vi "Main.vi"() -> ()   [LabVIEW 2018]
doc: "The myRIO Project template acquires acceleration data from the onboard accelerometer and displays the changes of acceleration values in a waveform chart."
uses:
  <vilib>/Platform/TimedLoop/XDataNode/timing_clust.ctl
  <vilib>/Platform/TimedLoop/XDataNode/nitl_modes.ctl
  <vilib>/Platform/TimedLoop/XDataNode/wakeup.ctl
  <vilib>/myRIO/Instrument Drivers/Onboard IO/DIO/typedefs/DIO Reference.ctl
  <vilib>/myRIO/Common/Instrument Driver Framework/Utilities/typedefs/myRIO Generic Hardware Reference.ctl
  <vilib>/myRIO/Common/Instrument Driver Framework/Utilities/typedefs/Hardware Version Enum.ctl
  <vilib>/myRIO/Common/Instrument Driver Framework/Utilities/typedefs/myRIO v1.0 Reference.ctl
  <vilib>/myRIO/Common/Instrument Driver Framework/Utilities/typedefs/Generic FPGA Reference.ctl
  <vilib>/myRIO/Common/Instrument Driver Framework/myRIO v1.0/DIO/typedefs/DIO Channels List.ctl
  <vilib>/myRIO/Common/Instrument Driver Framework/myRIO v1.0/DIO/typedefs/DIO Channels Enum.ctl
  <vilib>/userdefined/High Color/nirio_resource_hc.ctl
  <vilib>/myRIO/Instrument Drivers/Onboard IO/AI/typedefs/AI Reference.ctl
  <vilib>/myRIO/Common/Instrument Driver Framework/myRIO v1.0/AI/typedefs/AI Channels List.ctl
  <vilib>/myRIO/Common/Instrument Driver Framework/myRIO v1.0/AI/typedefs/AI Channels Enum.ctl
  <vilib>/myRIO/Common/Instrument Driver Framework/Utilities/typedefs/Analog Scaling Constants List.ctl
  <vilib>/myRIO/Common/Instrument Driver Framework/Utilities/typedefs/Analog Scaling Constants.ctl
  <vilib>/myRIO/Instrument Drivers/Onboard IO/AO/typedefs/AO Reference.ctl
  <vilib>/myRIO/Common/Instrument Driver Framework/myRIO v1.0/AO/typedefs/AO Channels List.ctl
  <vilib>/myRIO/Common/Instrument Driver Framework/myRIO v1.0/AO/typedefs/AO Channels Enum.ctl
  <vilib>/myRIO/Common/Instrument Driver Framework/Utilities/vis/Is FPGA Ref Available.vi
  <vilib>/myRIO/Common/Instrument Driver Framework/myRIO v1.0/DIO/vis/myRIO v1.1 Open DIO.vi
  <vilib>/myRIO/Instrument Drivers/Onboard IO/DIO/vis/Read.vi
  <vilib>/myRIO/Instrument Drivers/Onboard IO/DIO/vis/Write.vi
  <vilib>/myRIO/Common/Instrument Driver Framework/myRIO v1.0/AI/vis/myRIO v1.1 Open AI.vi
  <vilib>/myRIO/Instrument Drivers/Onboard IO/AI/vis/Read.vi
  <vilib>/myRIO/Common/Instrument Driver Framework/myRIO v1.0/AO/vis/myRIO v1.1 Open AO.vi
  <vilib>/myRIO/Instrument Drivers/Onboard IO/AO/vis/Write.vi
  <vilib>/myRIO/Common/Instrument Driver Framework/Utilities/vis/Validate Channels.vi
  <vilib>/myRIO/Common/Instrument Driver Framework/myRIO v1.0/DIO/vis/myRIO v1.0 Reserve DIO.vi
  <vilib>/myRIO/Common/Instrument Driver Framework/myRIO v1.0/AI/vis/myRIO v1.0 Reserve AI.vi
  <vilib>/myRIO/Common/Instrument Driver Framework/myRIO v1.0/AO/vis/myRIO v1.0 Reserve AO.vi
  <vilib>/myRIO/Common/Instrument Driver Framework/myRIO v1.0/Resource Manager/vis/myRIO v1.0 Reserve Channel List.vi
  <vilib>/myRIO/Common/Instrument Driver Framework/myRIO v1.0/DIO/vis/myRIO v1.0 Build MUX Configuration DIO.vi
  <vilib>/myRIO/Common/Instrument Driver Framework/myRIO v1.0/AI/vis/myRIO v1.0 Build MUX Configuration AI.vi
  <vilib>/myRIO/Common/Instrument Driver Framework/myRIO v1.0/AO/vis/myRIO v1.0 Build MUX Configuration AO.vi
  <vilib>/myRIO/Common/Instrument Driver Framework/myRIO v1.0/Resource Manager/vis/myRIO v1.0 Reserve Channel.vi
  <vilib>/myRIO/Common/Instrument Driver Framework/myRIO v1.0/Resource Manager/vis/myRIO v1.0 Unreserve Channel.vi
  <vilib>/myRIO/Common/Instrument Driver Framework/myRIO v1.0/Resource Manager/vis/myRIO v1.0 Create Configuration List.vi
  <vilib>/myRIO/Common/Instrument Driver Framework/myRIO v1.0/Resource Manager/vis/myRIO v1.0 Build Mutex Name.vi
  <vilib>/Utility/VariantDataType/GetNumericInfo.vi
  <vilib>/Utility/error.llb/Error Cluster From Error Code.vi
  <vilib>/myRIO/Common/Instrument Driver Framework/myRIO v1.0/myRIO v1.1 Open.vi
  <vilib>/myRIO/Common/Instrument Driver Framework/Utilities/vis/IO Manager.vi
  <vilib>/myRIO/Common/Instrument Driver Framework/Utilities/vis/Configuration Manager.vi
  <vilib>/myRIO/Common/Instrument Driver Framework/myRIO v1.0/Resource Manager/vis/myRIO v1.0 Configure IO.vi
  <vilib>/myRIO/Common/Instrument Driver Framework/myRIO v1.0/myRIO v1.0 Close.vi
  <vilib>/myRIO/Common/Instrument Driver Framework/myRIO v1.0/DIO/vis/myRIO v1.0 Write DIO.vi
  <vilib>/myRIO/Common/Instrument Driver Framework/myRIO v1.0/AI/vis/myRIO v1.0 Get Scaling Constants AI.vi
  <vilib>/myRIO/Common/Instrument Driver Framework/myRIO v1.0/AI/vis/myRIO v1.0 Read AI.vi
  <vilib>/functionblocks/Bistables/SR Bistable/SR Bistable.vi
  <vilib>/myRIO/Common/Instrument Driver Framework/myRIO v1.0/AO/vis/myRIO v1.0 Get Scaling Constants AO.vi
  <vilib>/myRIO/Common/Instrument Driver Framework/myRIO v1.0/AO/vis/myRIO v1.0 Write AO.vi
  <vilib>/functionblocks/Counter/Pulse Timer/Pulse Timer.vi
  <vilib>/myRIO/Common/Instrument Driver Framework/myRIO v1.0/DIO/vis/myRIO v1.0 Read DIO.vi
  <vilib>/myRIO/Express VI/Onboard IO/DO/DO Express VI.xnode
  <vilib>/myRIO/Instrument Drivers/Onboard IO/DIO/vis/myRIO DIO Open.xnode
  <vilib>/Platform/TimedLoop/XDataNode/XDataNode.xnode
  <vilib>/myRIO/Express VI/Onboard IO/AI/AI Express VI.xnode
  <vilib>/myRIO/Instrument Drivers/Onboard IO/AI/vis/myRIO AI Open.xnode
  <vilib>/functionblocks/FB Core/FB Core.xnode
  <vilib>/myRIO/Express VI/Onboard Devices/LED/LED Express VI.xnode
  <vilib>/myRIO/Express VI/Onboard IO/AO/AO Express VI.xnode
  <vilib>/myRIO/Instrument Drivers/Onboard IO/AO/vis/myRIO AO Open.xnode
  <vilib>/myRIO/Express VI/Onboard IO/DI/DI Express VI.xnode
  <vilib>/myRIO/Express VI/Onboard Devices/Button/Button Express VI.xnode
  <vilib>/myRIO/Instrument Drivers/Onboard IO/DIO/DIO.lvlib
  <vilib>/myRIO/Instrument Drivers/Onboard IO/AI/AI.lvlib
  <vilib>/myRIO/Instrument Drivers/Onboard IO/AO/AO.lvlib
  <vilib>/functionblocks/NI_FunctionBlock Libraries.lvlib
  <vilib>/Platform/TimedLoop/XDataNode/XDNodeRunTimeDep.lvlib
panel:
  out "Pump out":bool
  out "RTD Status LED":bool
  out "RFE Indicator":bool
  out "AIR + Boolean":bool
  out "AIR +(A9)":dbl
  out "RTD Button":bool
  out "RTD Brake":bool
  out "EN Indicator":bool
  out "RTD Buzzer":bool
  in  "Buzzer test":bool
  in  "RTD Brake Test":bool
  in  "RFE  Test":bool
  in  "EN Test":bool
  out "APPS1 (V) Input (B/AI0 (Pin 3))":dbl
  out "APPS2 Scaled Up (V)":dbl
  out "APPS1 Scaled Up (V)":dbl
  out "APPS2 (V) Input (B/AI1 (Pin 5))":dbl
  out "APPS fault":bool
  out "APPS2 %":dbl
  out "APPS1 %":dbl
  out "APPS Output (V)":dbl
  out "APPS output %":dbl
  out "Accelaration":dbl(knob) scale=0.0..100.0
  out "APPS1":dbl(knob) scale=0.0..100.0
  out "APPS2":dbl(knob) scale=0.0..100.0
  out "APPS pedal travel %":dbl
  out "RTD Brake 2":bool
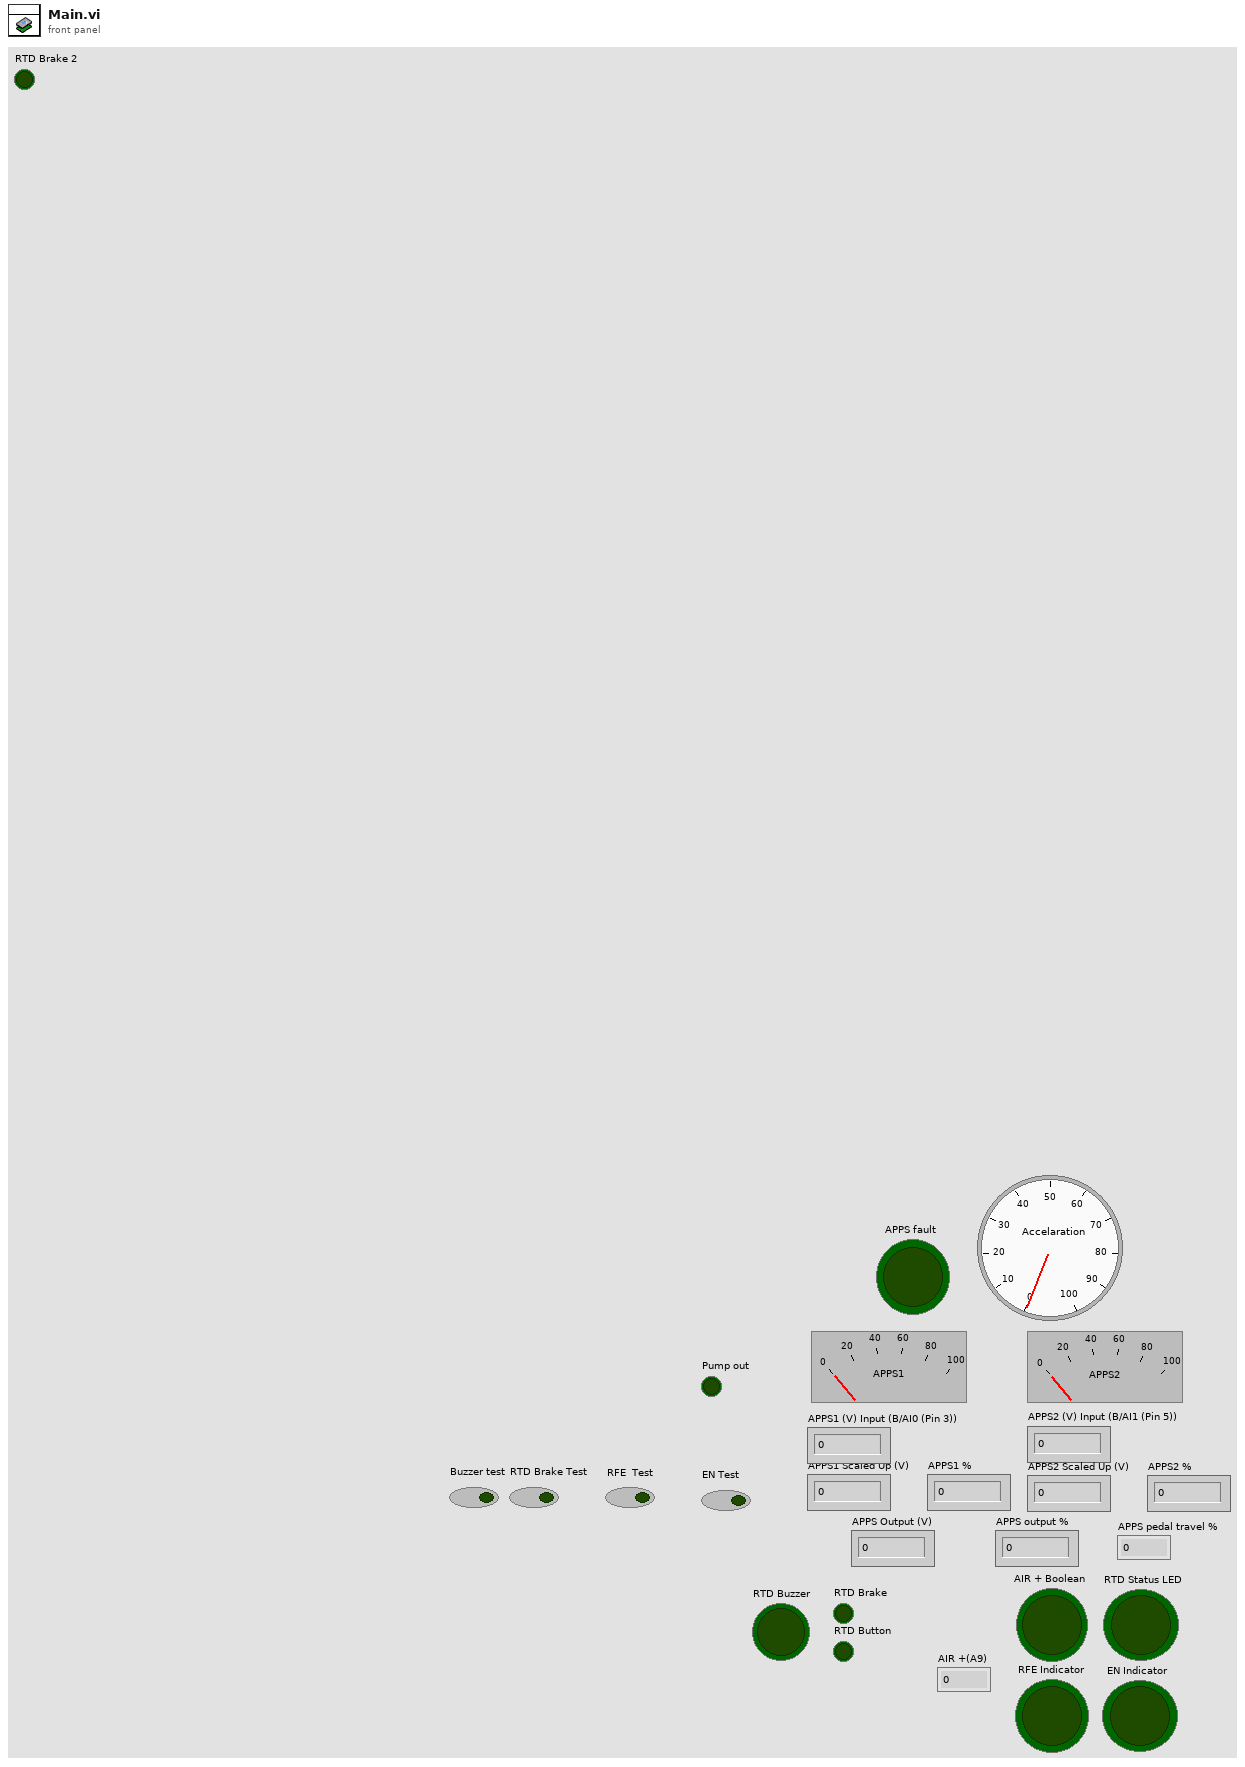
[diagram p1: front panel]
types:
  T1 = typedef "XDNodeRunTimeDep.lvlib/timing_clust.ctl" = cluster{"Expected End [f-1]":u64, "Actual End [f-1]":u64, "Finished Late? [f-1]":bool, "Expected End [i-1]":u64, "Actual End [i-1]":u64, "Finished Late? [i-1]":bool, "Expected Start [i]":u64, "Actual Start [i]":u64, "Expected Start [f]":u64, "Actual Start [f]":u64, "Source Name":string, "Structure Name":string, "Period":i64, "Deadline":i64, "Offset":i64, "Start":i64, "Priority":i32, "Timeout":i32, "Mode":T2, "Wakeup Reason":T3, "Error":errorcluster, "Source Type":string, "Secondary Source Type":string, "Global End Time":u64, "Global Start Time":u64, "Frame Duration":u64, "Iteration Duration":u64, "Assigned CPU":i32, "I/O Scan Engine Mode":u32}
  T2 = typedef "XDNodeRunTimeDep.lvlib/nitl_modes.ctl" = enum32{"No Change", "Process missed periods, maintain original phase", "Discard missed periods, maintain original phase", "Process missed periods, ignore original phase", "Discard missed periods, ignore original phase"}
  T3 = typedef "XDNodeRunTimeDep.lvlib/wakeup.ctl" = enum32{"Normal", "Aborted", "Asynchronous wakeup", "Timing source error", "Timed loop error", "Timeout"}
  T4 = typedef "DIO.lvlib/DIO Reference.ctl" = cluster{"myRIO Reference":T5, "DIO Channels List":T9}
  T5 = typedef "myRIO Generic Hardware Reference.ctl" = cluster{"myRIO Model":T6, "myRIO Hardware Reference":T7}
  T6 = typedef "Hardware Version Enum.ctl" = enum16{"Unknown", "myRIO-1900", "myRIO-1950", "roboRIO", "NI ELVIS RIO CM", "ELVIS III"}
  T7 = typedef "myRIO v1.0 Reference.ctl" = cluster{"Generic FPGA Reference":T8, "Allow multiple opens":bool}
  T8 = typedef "Generic FPGA Reference.ctl" = refnum<k20>
  T9 = typedef "DIO Channels List.ctl" = T10[]
  T10 = typedef "DIO Channels Enum.ctl" = enum16{"Not Connected", "C/DIO0", "C/DIO1", "C/DIO2", "C/DIO3", "C/DIO4", "C/DIO5", "C/DIO6", "C/DIO7", "A/DIO0", "A/DIO1", "A/DIO2", "A/DIO3", "A/DIO4", "A/DIO5", "A/DIO6", "A/DIO7", "A/DIO8", "A/DIO9", "A/DIO10", "A/DIO11", "A/DIO12", "A/DIO13", "A/DIO14", "A/DIO15", "A/DIO16", "A/DIO17", "A/DIO18", "A/DIO19", "B/DIO0", "B/DIO1", "B/DIO2", "B/DIO3", "B/DIO4", "B/DIO5", "B/DIO6", "B/DIO7", "B/DIO8", "B/DIO9", "B/DIO10", "B/DIO11", "B/DIO12", "B/DIO13", "B/DIO14", "B/DIO15", "B/DIO16", "B/DIO17", "B/DIO18", "B/DIO19", "LED0", "LED1", "LED2", "LED3", "Button0", "DIO/DIO0", "DIO/DIO1", "DIO/DIO2", "DIO/DIO3", "DIO/DIO4", "DIO/DIO5", "DIO/DIO6", "DIO/DIO7", "DIO/DIO8", "DIO/DIO9", "SPI/CS0", "SPI/CS1", "SPI/CS2", "SPI/CS3", "LED RADIO (Green)", "LED RADIO (Red)", "LED COMM (Green)", "LED COMM (Red)", "LED MODE (Green)", "LED MODE (Red)"}
  T11 = typedef "nirio_resource_hc.ctl" = tag
  T12 = typedef "AO.lvlib/AO Reference.ctl" = cluster{"myRIO Reference":T5, "AO Channel List":T13, "AO Scaling Constant List":T15}
  T13 = typedef "AO Channels List.ctl" = T14[]
  T14 = typedef "AO Channels Enum.ctl" = enum16{"Not Connected", "AudioOut/Left", "AudioOut/Right", "C/AO0", "C/AO1", "A/AO0", "A/AO1", "B/AO0", "B/AO1"}
  T15 = typedef "Analog Scaling Constants List.ctl" = T16[]
  T16 = typedef "Analog Scaling Constants.ctl" = cluster{"LSB Weight (Volts)":dbl, "Offset (Volts)":dbl, "Signed?":bool}
  T17 = typedef "AI.lvlib/AI Reference.ctl" = cluster{"myRIO Reference":T5, "AI Channels List":T18, "AI Scaling Constants List":T15}
  T18 = typedef "AI Channels List.ctl" = T19[]
  T19 = typedef "AI Channels Enum.ctl" = enum16{"Not Connected", "AudioIn/Left", "AudioIn/Right", "C/AI0", "C/AI1", "A/AI0", "A/AI1", "A/AI2", "A/AI3", "A/AI4", "A/AI5", "A/AI6", "A/AI7", "B/AI0", "B/AI1", "B/AI2", "B/AI3", "B/AI4", "B/AI5", "B/AI6", "B/AI7", "AI/AI0", "AI/AI1", "AI/AI2", "AI/AI3", "A/AI0 (DIFF)", "A/AI1 (DIFF)", "A/AI2 (DIFF)", "A/AI3 (DIFF)", "B/AI0 (DIFF)", "B/AI1 (DIFF)", "B/AI2 (DIFF)", "B/AI3 (DIFF)"}
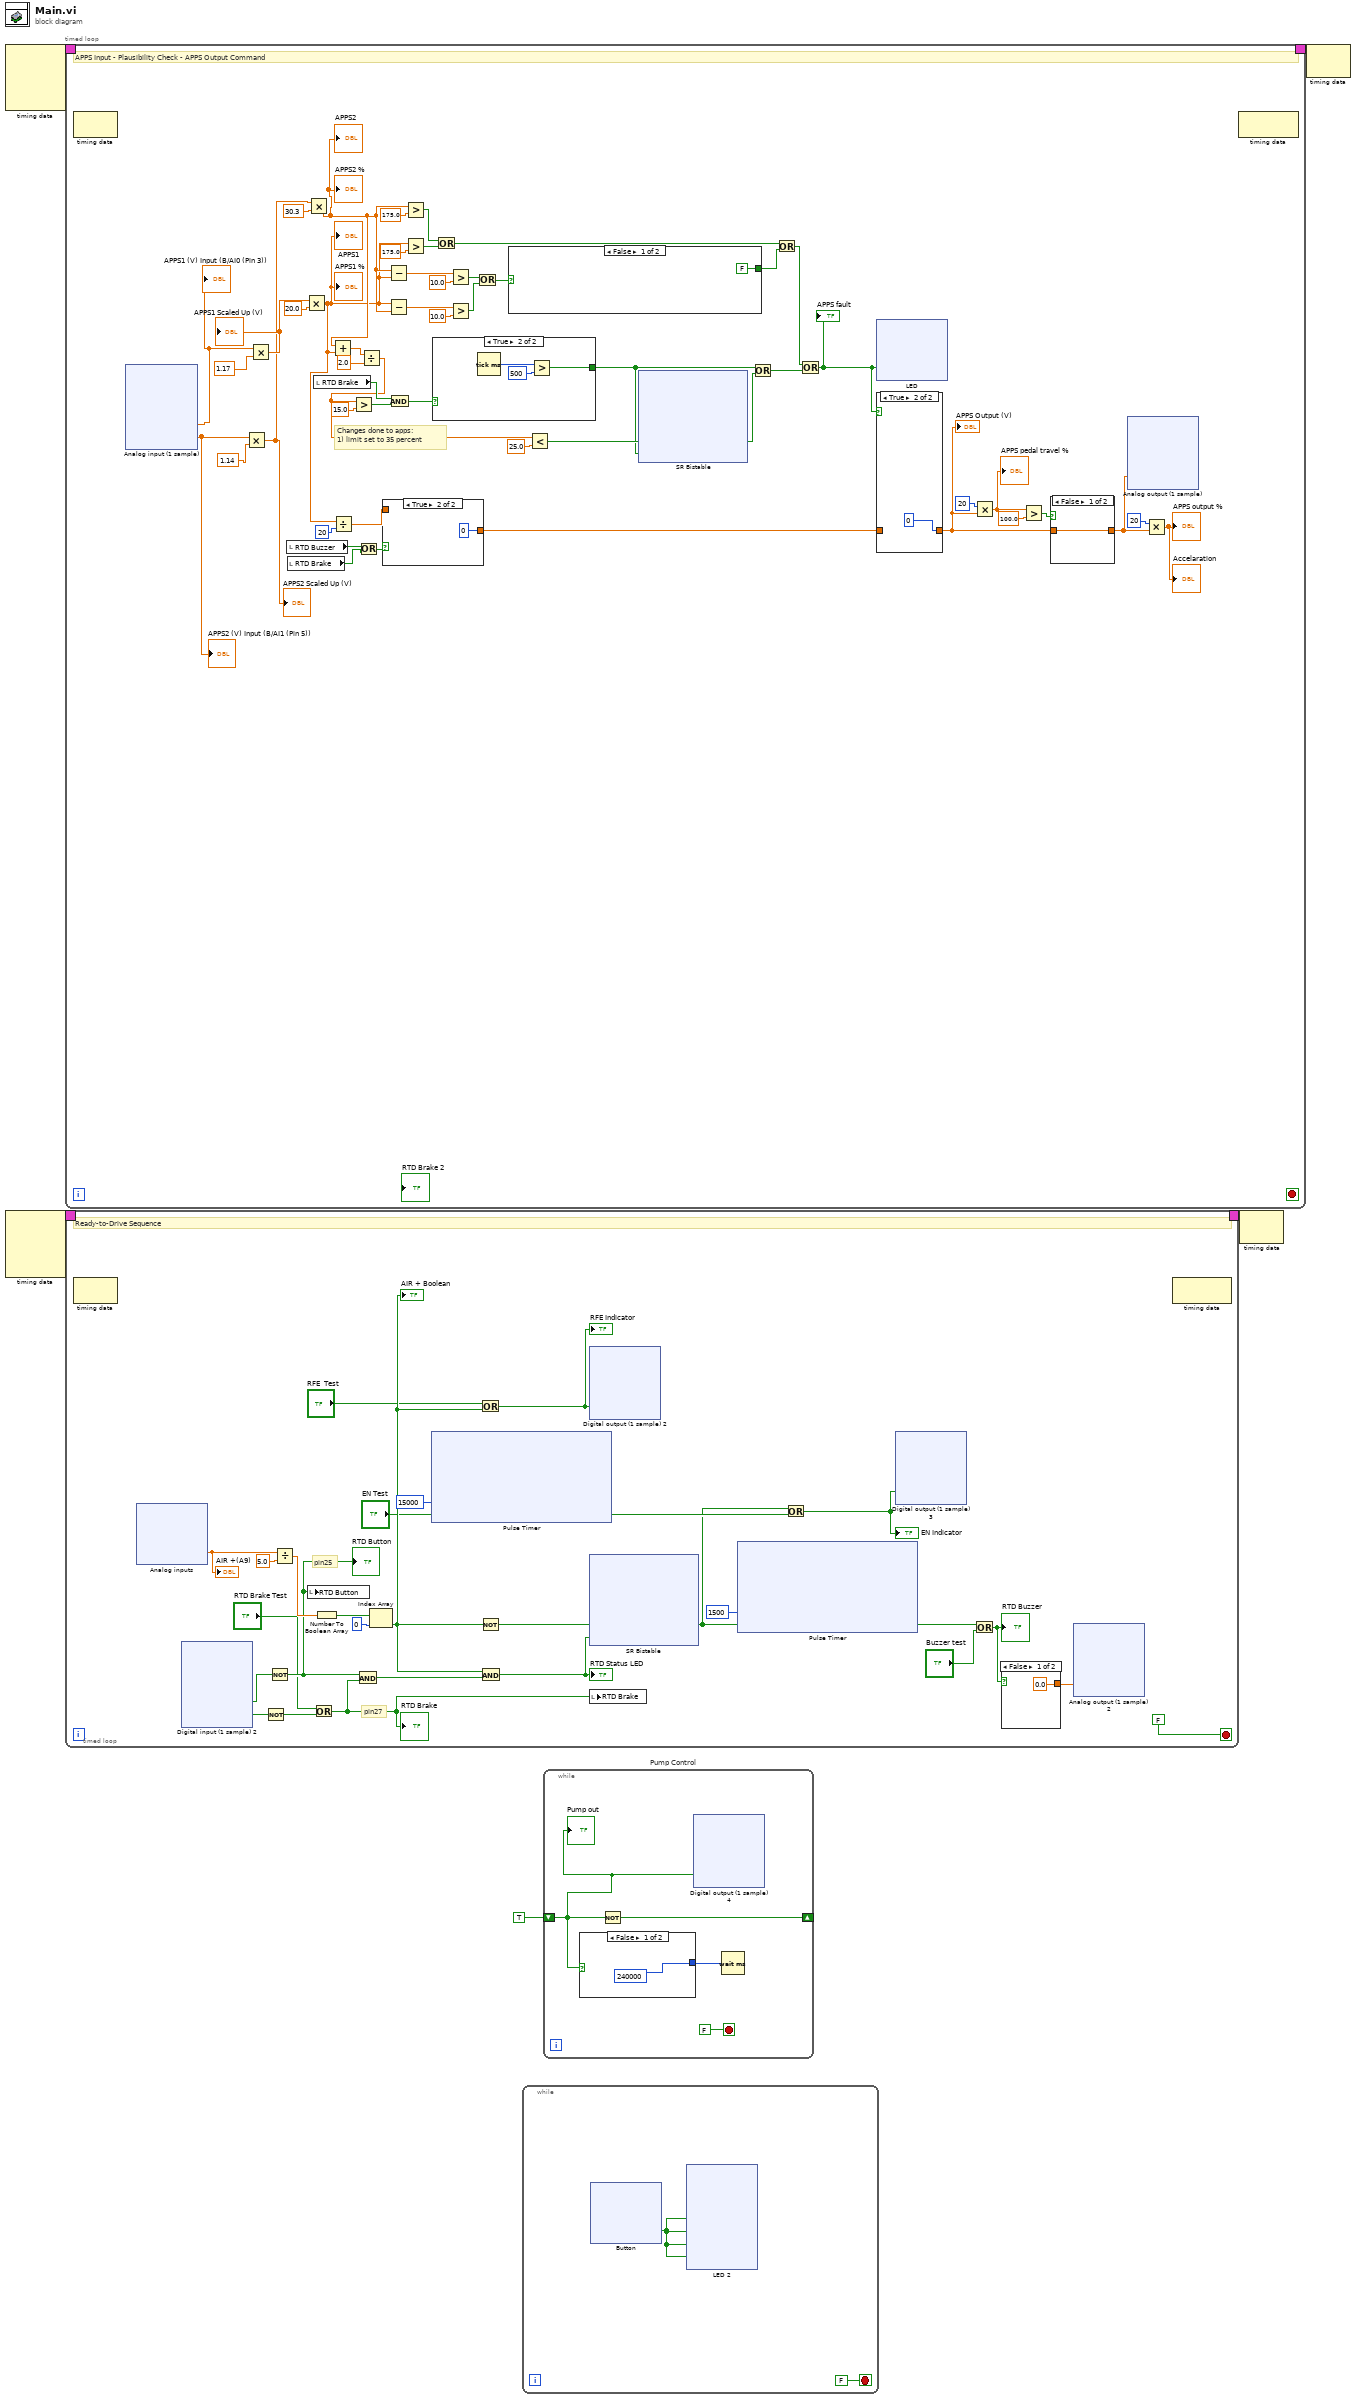
[diagram p0: block diagram]
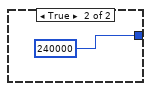
[diagram p2: hidden frame]
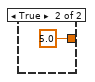
[diagram p3: hidden frame]
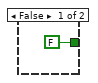
[diagram p4: hidden frame]
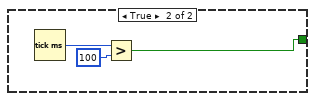
[diagram p5: hidden frame]
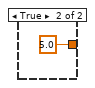
[diagram p7: hidden frame]
diagram:
  n1 = node-c288() -> (w5:T1)  [unwired: 4 in]
  n2 = node-c288() -> (w3:T1)  [unwired: 4 in]
  n3 = timed-loop {
    timing: w5 -> [_]
    timing-out: [_] -> w4
    stop <- _ stop-if-true
    # "Changes done to apps:\n1) limit set to 35 percent"
    # "APPS Input - Plausibility Check - APPS Output Command"
    n4 = node-c288() -> ()  [unwired: 1 in, 1 out]
    n5 = xnode "Analog input (1 sample)"() -> ("APPS 1 Input (B/AI0 (Pin 3))"=w8:dbl, "APPS 2 Input (B/AI1 (Pin 5))"=w14:dbl)  [unwired: 1 in, 1 out]
    "APPS1 (V) Input (B/AI0 (Pin 3))" <- w8
    "APPS2 (V) Input (B/AI1 (Pin 5))" <- w14
    n6 = Multiply(x=w14, y=1.14) -> (x*y=w7:dbl)
    "APPS2 Scaled Up (V)" <- w7
    n7 = Multiply(x=w8, y=1.17) -> (x*y=w12:dbl)
    "APPS1 Scaled Up (V)" <- w12
    n8 = local read "RTD Buzzer"() -> (w9:bool)
    n9 = local read "RTD Brake"() -> (w10:bool)
    n10 = Multiply(x=w12, y=20.0) -> (x*y=w17:dbl)
    "APPS1 %" <- w17
    "APPS1" <- w17
    n11 = Multiply(x=w7, y=30.3) -> (x*y=w18:dbl)
    "APPS2 %" <- w18
    "APPS2" <- w18
    n12 = local read "RTD Brake"() -> (w28:bool)
    n13 = Add(x=w18, y=w17) -> (x+y=w21:dbl)
    n14 = Divide(x=w17, y=20) -> (x/y=w16:dbl)
    n15 = Or(x=w9, y=w10) -> (x .or. y?=w11:bool)
    n16 = Divide(x=w21, y=2.0) -> (x/y=w19:dbl)
    n17 = Greater?(x=w19, y=15.0) -> (0:w41:bool)
    n18 = case shown="True" w11 {
      tunnel: [w109 0] -> w37
      tunnel: w16 -> [w109 _]
      frame False {
      }
      frame True {
      }
    }
    n19 = Subtract(x=w18, y=w17) -> (x-y=w54:dbl)
    n20 = Subtract(x=w17, y=w18) -> (x-y=w43:dbl)
    n21 = And(x=w28, y=w41) -> (x .and. y?=w24:bool)
    n22 = Greater?(x=w18, y=175.0) -> (0:w51:bool)
    n23 = Greater?(x=w17, y=175.0) -> (0:w50:bool)
    n24 = case shown="True" w24 {
      tunnel: [FALSE w60] -> w23
      frame False {
      }
      frame True {
        n25 = Tick Count (ms)() -> (millisecond timer value=w62:u32)
        n26 = Greater?(x=w62, y=u32 500) -> (0:w60:bool)
      }
    }
    n27 = Or(x=w51, y=w50) -> (x .or. y?=w49:bool)
    n28 = Greater?(x=w54, y=10.0) -> (0:w55:bool)
    n29 = Greater?(x=w43, y=10.0) -> (0:w44:bool)
    n30 = Or(x=w55, y=w44) -> (x .or. y?=w32:bool)
    n31 = case shown="False" w32 {
      tunnel: [FALSE w106] -> w31
      frame False {
      }
      frame True {
        n32 = Tick Count (ms)() -> (millisecond timer value=w108:u32)
        n33 = Greater?(x=w108, y=u32 100) -> (0:w106:bool)
      }
    }
    n34 = Less?(x=w19, y=25.0) -> (x < y?=w29:bool)
    n35 = xnode "SR Bistable"("reset"=w29, "set"=w23) -> ("output"=w30:bool)  [unwired: 1 in, 1 out]
    n36 = Or(x=w23, y=w30) -> (x .or. y?=w26:bool)
    n37 = Or(x=w49, y=w31) -> (x .or. y?=w27:bool)
    n38 = Or(x=w27, y=w26) -> (x .or. y?=w25:bool)
    "APPS fault" <- w25
    n39 = xnode "LED"("LED0"=w25) -> ()  [unwired: 1 in, 1 out]
    n40 = case shown="True" w25 {
      tunnel: w37 -> [w113 _]
      tunnel: [w113 0] -> w36
      frame False {
      }
      frame True {
      }
    }
    "APPS Output (V)" <- w36
    n41 = Multiply(x=20, y=w36) -> (x*y=w22:dbl)
    "APPS pedal travel %" <- w22
    n42 = Greater?(x=w22, y=100.0) -> (0:w38:bool)
    n43 = case shown="False" w38 {
      tunnel: [w111 5.0 ("APPS output %")] -> w34
      tunnel: w36 -> [w111 _]
      frame False {
      }
      frame True {
      }
    }
    n44 = xnode "Analog output (1 sample)"("APPS Output (B/AO0 (Pin 2))"=w34) -> ()  [unwired: 1 in, 1 out]
    n45 = Multiply(x=20, y=w34) -> (x*y=→"APPS output %" →"Accelaration":dbl)
    n46 = node-c288() -> ()  [unwired: 1 in, 1 out]
  }
  n47 = timed-loop {
    timing: w3 -> [_]
    timing-out: [_] -> w2
    stop <- FALSE stop-if-true
    # "pin27"
    # "pin25"
    # "Ready-to-Drive Sequence"
    n48 = node-c288() -> ()  [unwired: 1 in, 1 out]
    n49 = xnode "Analog inputs"() -> ("AIR + (B/AI2 (Pin 7))"=w247:dbl)  [unwired: 1 in, 1 out]
    "AIR +(A9)" <- w247
    n50 = xnode "Digital input (1 sample) 2"() -> ("RTD Button (B/DIO2 (Pin 15))"=w246:bool, "RTD Brake (B/DIO3 (Pin 17))"=w245:bool)  [unwired: 1 in, 1 out]
    n51 = Not(x=w245) -> (.not. x?=w239:bool)
    n52 = Not(x=w246) -> (.not. x?=w243:bool)
    "RTD Button" <- w243
    n53 = Divide(x=w247, y=5.0) -> (x/y=w251:dbl)
    n54 = local write "RTD Button"(w243) -> ()
    n55 = Or(x="RTD Brake Test", y=w239) -> (x .or. y?=w238:bool)
    "RTD Brake" <- w238
    n56 = Number To Boolean Array(number=w251) -> (Boolean array=w252:bool[])
    n57 = And(x=w243, y=w238) -> (x .and. y?=w248:bool)
    n58 = Index Array(array=w252, index=0) -> (element=w237:bool)
    "AIR + Boolean" <- w237
    n59 = xnode "Pulse Timer"("preset time (ms)"=15000, "input"="EN Test") -> ("output"=w233:bool)  [unwired: 1 in, 2 out]
    n60 = Or(x="RFE  Test", y=w237) -> (x .or. y?=w236:bool)
    "RFE Indicator" <- w236
    n61 = Not(x=w237) -> (.not. x?=w241:bool)
    n62 = And(x=w237, y=w248) -> (x .and. y?=w242:bool)
    "RTD Status LED" <- w242
    n63 = xnode "Digital output (1 sample) 2"("RFE (B/DIO0 (Pin 11))"=w236) -> ()  [unwired: 1 in, 1 out]
    n64 = xnode "SR Bistable"("reset"=w241, "set"=w242) -> ("output"=w230:bool)  [unwired: 1 in, 1 out]
    n65 = local write "RTD Brake"(w238) -> ()
    n66 = xnode "Pulse Timer"("preset time (ms)"=1500, "input"=w230) -> ("output"=w228:bool)  [unwired: 1 in, 2 out]
    n67 = Or(x=w230, y=w233) -> (x .or. y?=w232:bool)
    "EN Indicator" <- w232
    n68 = xnode "Digital output (1 sample) 3"("EN (B/DIO1 (Pin 13))"=w232) -> ()  [unwired: 1 in, 1 out]
    n69 = Or(x=w228, y="Buzzer test") -> (x .or. y?=w227:bool)
    "RTD Buzzer" <- w227
    n70 = case shown="False" w227 {
      tunnel: [0.0 ("y") 5.0 ("y")] -> w244
      frame False {
      }
      frame True {
      }
    }
    n71 = xnode "Analog output (1 sample) 2"("RTD - Buzzer (B/AO1 (Pin 4))"=w244) -> ()  [unwired: 1 in, 1 out]
    n72 = node-c288() -> ()  [unwired: 1 in, 1 out]
  }
  n73 = while {
    stop <- FALSE stop-if-true
    n74 = xnode "Button"() -> ("Value"=w563:bool)  [unwired: 1 in, 1 out]
    n75 = xnode "LED 2"("LED0"=w563, "LED1"=w563, "LED2"=w563, "LED3"=w563) -> ()  [unwired: 1 in, 1 out]
  }
  n76 = while "Pump Control" {
    shift-right: [w641] -> _
    shift-left: TRUE -> [w638]
    stop <- FALSE stop-if-true
    n77 = case shown="False" w638 {
      tunnel: [240000 240000] -> w640
      frame False {
      }
      frame True {
      }
    }
    n78 = Not(x=w638) -> (.not. x?=w641:bool)
    n79 = xnode "Digital output (1 sample) 4"("Pump out (B/DIO8 (Pin 27))"=w638) -> ()  [unwired: 1 in, 1 out]
    n80 = Wait (ms)(milliseconds to wait=w640) -> ()  [unwired: 1 out]
    "Pump out" <- w638
  }
  n81 = node-c288(w2) -> ()  [unwired: 1 out]
  n82 = node-c288(w4) -> ()  [unwired: 1 out]
